vi "UniCyRO Environment Simulator.vi"() -> ()   [LabVIEW 2012]
doc: "This VI starts and stops the environment simulator and serves as the master VI for your simulation code. Open and run this VI to display the environment simulator, or open the block diagram to view or modify simulation code."
uses:
  Model/UniCyRO/UniCyRO_Host_Sim.lvclass
  <vilib>/robotics/Simulator/NI_Robotics_Simulator.lvlib
panel:
  in  "Torsion Motor ccw velocity (rad/s)":dbl(slide) scale=-10.0..10.0
  in  "Drive Motor ccw velocity (rad/s)":dbl(slide) scale=-10.0..10.0
  in  "Gyro Motor ccw velocity (rad/s)":dbl(slide) scale=-10.0..10.0
  in  "manifest filename":string="UniCyRO Environment Simulator.xml"
  in  "stop":bool
  # "* Press the Run button to display the Robotics Environment Simulator.\n* Select Window>>Show Block Diagram or press <Ctrl-E> to view the block diagram, where you can add or modify simulation code. Add controls and indicators to the front panel of this VI to pass data into and out of the simulation code.\n* The manifest file must exist in same directory as the .lvproj file."
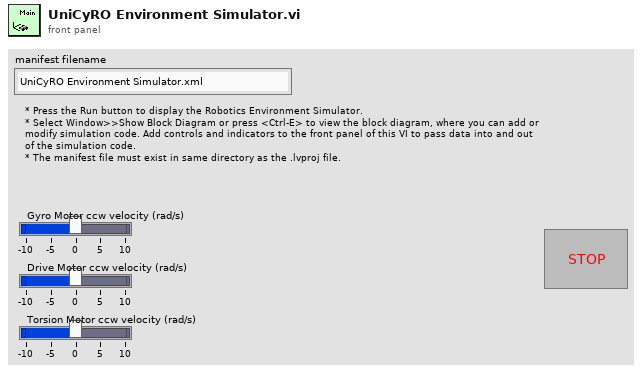
[diagram p1: front panel]
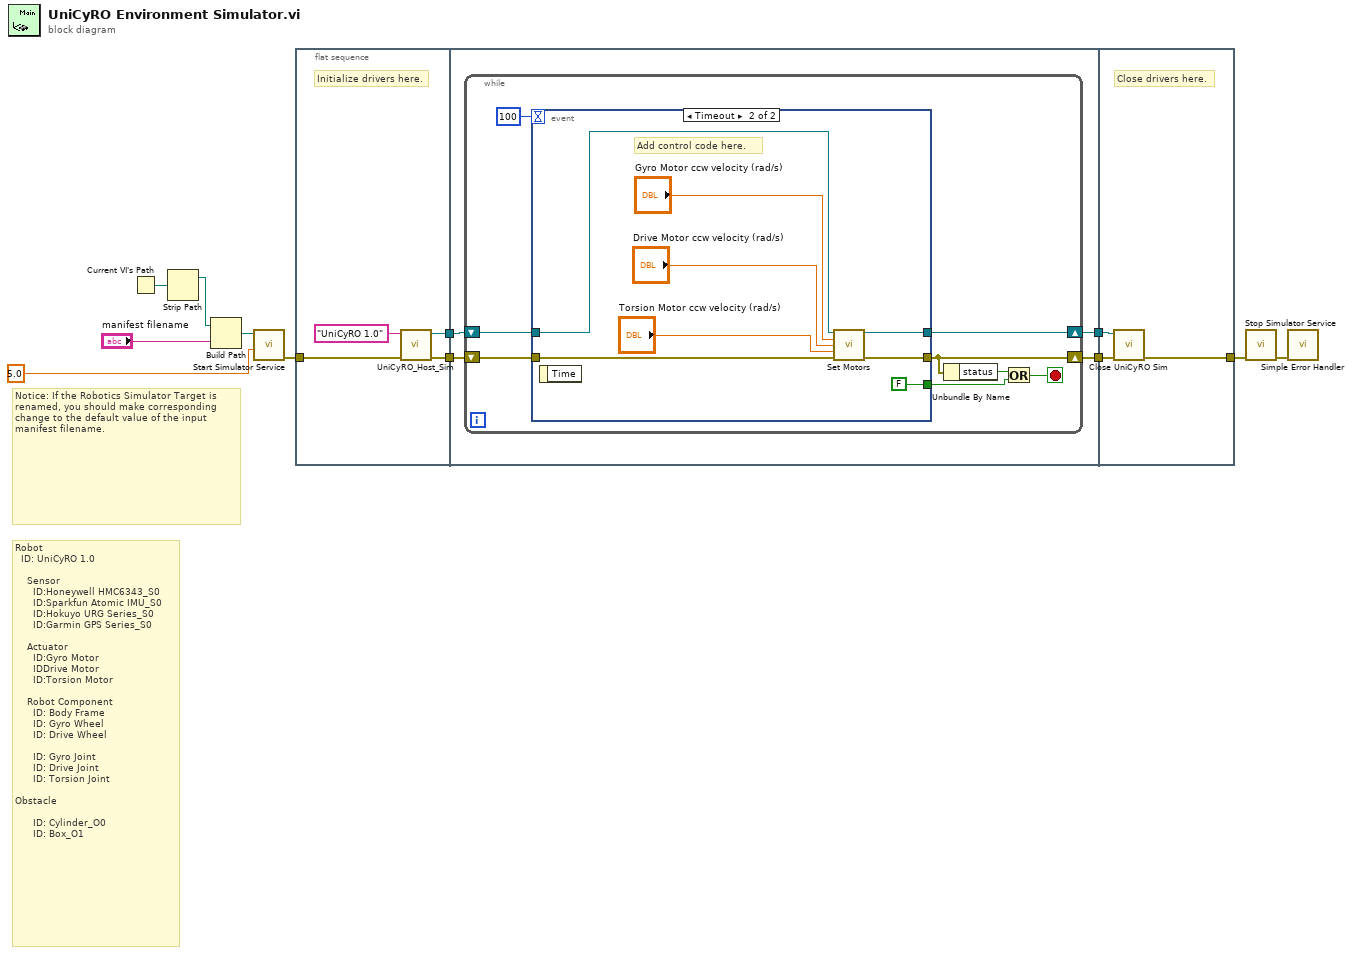
[diagram p0: block diagram]
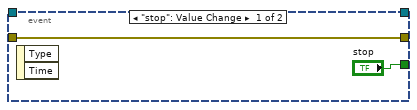
[diagram p2: hidden frame]
diagram:
  # "Robot\n\t\tID: UniCyRO 1.0\n\n\t\t\t\tSensor\n\t\t\t\t\t\tID:Honeywell HMC6343_S0\n      ID:Sparkfun Atomic IMU_S0\n      ID:Hokuyo URG Series_S0\n      ID:Garmin GPS Series_S0\n\n\t\t\t\tActuator\n      ID:Gyro Motor\n      IDDrive Motor\n      ID:Torsion Motor\n\n\t\t\t\tRobot Component\n\t\t\t\t\t\tID: Body Frame\n\t\t\t\t\t\tID: Gyro Wheel\n\t\t\t\t\t\tID: Drive Wheel\n\n\t\t\t\t\t\tID: Gyro Joint\n\t\t\t\t\t\tID: Drive Joint\n\t\t\t\t\t\tID: Torsion Joint\n\nObstacle\n\n      ID: Cylinder_O0\n      ID: Box_O1"
  # "Notice: If the Robotics Simulator Target is renamed, you should make corresponding change to the default value of the input manifest filename."
  n1 = Current VI's Path() -> (path=w10:path)
  n2 = Strip Path(path=w10) -> (stripped path=w9:path)  [unwired: 1 out]
  n3 = Build Path(base path=w9, name or relative path="manifest filename") -> (appended path=w8:path)
  n4 = call <vilib>:"Start Simulator Service.vi"("step size (ms)"=5.0 ("stepsize(ms)"), "manifest file"=w8) -> ("error out"=w5:errorcluster)  [unwired: 9 in]
  n5 = flat-sequence {
    tunnel: w5 -> [w16]
    tunnel: [w15] -> w4
    tunnel: [w13] -> w2
    tunnel: w4 -> [w19]
    tunnel: [w20] -> w3
    tunnel: w2 -> [w18]
    tunnel: [w17] -> w1
    tunnel: [w40] -> w11
    tunnel: w3 -> [w41]
    tunnel: w1 -> [w39]
    frame #0 {
      # "Initialize drivers here."
      n6 = call "UniCyRO_Host_Sim"("error in (no error)"=w16, "robot ID"="UniCyRO 1.0") -> ("error out"=w15:errorcluster, "UniCyRO_Host_Sim out"=w13:refnum<class "UniCyRO_Host_Sim.lvclass">)  [unwired: 8 in]
    }
    frame #1 {
      n7 = while {
        shift-right: [w24] -> w20
        shift-left: w19 -> [w27]
        shift-right: [w21] -> w17
        shift-left: w18 -> [w22]
        stop <- w25 stop-if-true
        n8 = event shown="[1] Timeout" {
          selector: _ -> [_ _]
          dyn-events: _ -> [_ _]
          timeout: 100 -> [_ _]
          tunnel: ["stop" FALSE ("stop")] -> w26
          tunnel: [w29 w34] -> w24
          tunnel: w27 -> [w29 w35]
          tunnel: w22 -> [_ w37]
          tunnel: [_ w36] -> w21
          event "stop": Value Change {
            n9 = event-data() -> ()  [unwired: 1 in, 2 out]
          }
          event Timeout {
            # "Add control code here."
            n10 = event-data() -> ()  [unwired: 1 in, 1 out]
            n11 = call "Set Motors.vi"("UniCyRO_Host_Sim in"=w37, "Gyro Motor ccw velocity (rad/s)"="Gyro Motor ccw velocity (rad/s)", "Drive Motor ccw velocity (rad/s)"="Drive Motor ccw velocity (rad/s)", "Torsion Motor ccw velocity (rad/s)"="Torsion Motor ccw velocity (rad/s)", "error in (no error)"=w35) -> ("UniCyRO_Host_Sim out"=w36:refnum<class "UniCyRO_Host_Sim.lvclass">, "error out"=w34:errorcluster)  [unwired: 9 in]
          }
        }
        n12 = Unbundle By Name(w24) -> ("status"=w23:bool)
        n13 = Or(x=w23, y=w26) -> (x .or. y?=w25:bool)
      }
    }
    frame #2 {
      # "Close drivers here."
      n14 = call "Close UniCyRO Sim.vi"("error in (no error)"=w41, "UniCyRO_Host_Sim in"=w39) -> ("error out"=w40:errorcluster)  [unwired: 9 in]
    }
  }
  n15 = call <vilib>:"Stop Simulator Service.vi"("error in (no error)"=w11) -> ("error out"=w6:errorcluster)  [unwired: 10 in]
  n16 = call <vilib>:"Simple Error Handler.vi"("error in (no error)"=w6) -> ()  [unwired: 4 in, 5 out]
